vi "Simple main.vi"() -> ()   [LabVIEW 2021]
doc: "Use this template to build a simple state machine design pattern. Each state executes code and determines which state to transition to."
uses:
  controls/Data.ctl
  controls/State.ctl
  <instrlib>/Lake Shore 350/Lake Shore 350.lvlib
  <instrlib>/Keithley 2450/Keithley 2450.lvlib
panel:
  in  "Two way":bool
  out "Since last point (s)":dbl caption="Elapsed Time (s)"
  in  "Data spacing":enum16{"Log", "Quadratic", "Cubic", "Linear"}(ring)
  in  "Time Target (s)":dbl=3600.0 format="%#_13g"
  in  "Number of points":i32=390
  out "Progress %":dbl(slide) caption="Horizontal Pointer Slide" scale=0.0..100.0
  out "Data":T1
  in  "Start point":dbl
  in  "End point":dbl
  in  "Use second SMUs":bool
  in  "Stop btn":bool
  in  "Start btn":bool
  in  "Instruments":T2 {"SMU 2"."Last updated" format="%<%H:%M:%S>T"; "SMU 1"."Last updated" format="%<%H:%M:%S>T"; "TC"."Last updated" format="%<%H:%M:%S>T"}
  in  "End btn":bool
  out "Actual temperature chart":dbl[](graph)
  out "Rezistance graph":cluster{dbl[], dbl[]}[](graph)
  out "Message logs":string[](array[string])
  # "T=1,6*exp(0,0135*n)     where n is N in <1,"
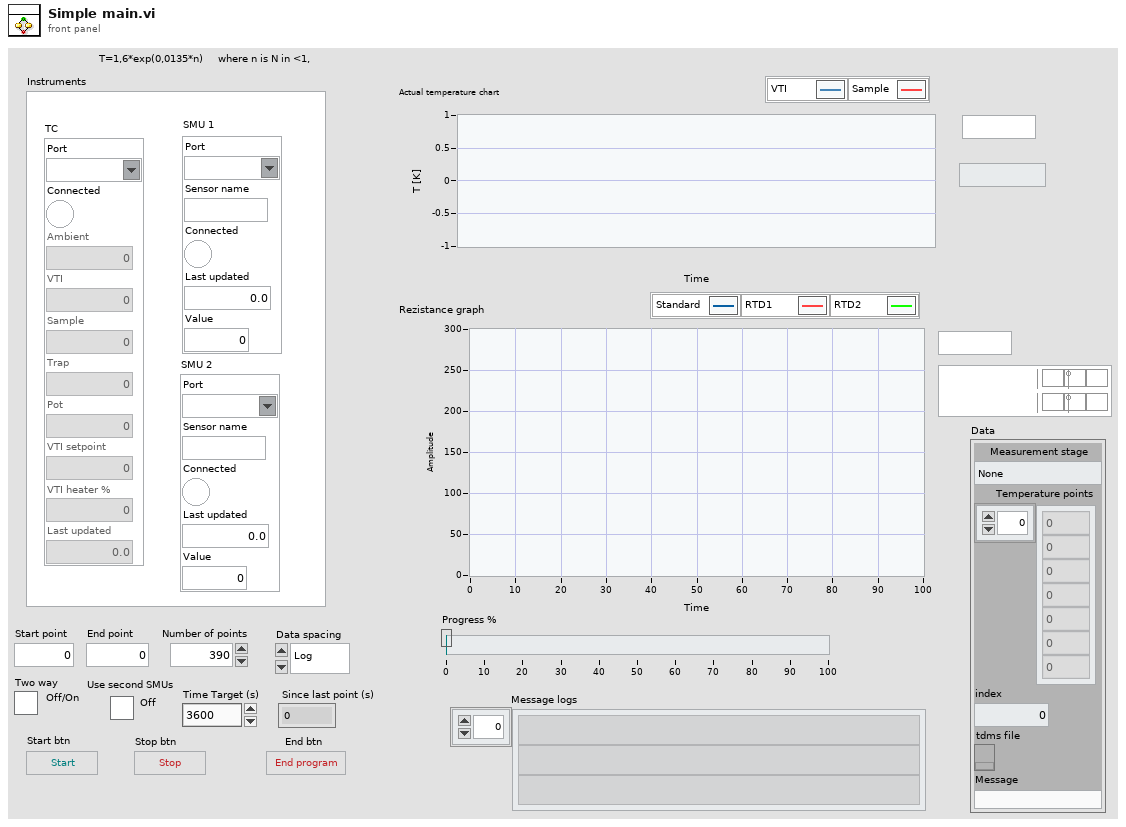
[diagram p1: front panel]
types:
  T1 = typedef "Data.ctl" = cluster{"Measurement stage":enum16{"None", "Wait to start", "Stage 1", "Interstage", "Stage 2", "Stopping"}, "Temperature points":dbl[], "index":i32, "tdms file":refnum<k34>, "Message":string}
  T2 = cluster{"TC":cluster{"Port":refnum<visa-resource-name>, "Connected":bool, "Ambient":dbl, "VTI":dbl, "Sample":dbl, "Trap":dbl, "Pot":dbl, "VTI setpoint":dbl, "VTI heater %":dbl, "Last updated":dbl}, "SMU 1":cluster{"Port":refnum<visa-resource-name>, "Sensor name":string, "Connected":bool, "Last updated":dbl, "Value":dbl}, "SMU 2":cluster{"Port":refnum<visa-resource-name>, "Sensor name":string, "Connected":bool, "Last updated":dbl, "Value":dbl}}
  T3 = typedef "State.ctl" = enum16{"Initialize", "Connect to TC", "Disconnect TC", "Connect to SMU", "Disconnect SMU ", "Set TC", "Read TC", "Set SMU", "Read SMU", "Wait for Event", "Start measurement", "Save datapoint", "End measurement", "Stop program"}
  T4 = enum16{"None", "Wait to start", "Stage 1", "Interstage", "Stage 2", "Stopping"}
  T5 = cluster{"Baud Rate":u32, "Parity":u16, "Data Bits":u16, "Stop Bits":u16, "Flow Control":u16}
  T6 = cluster{"Port":refnum<visa-resource-name>, "Sensor name":string, "Connected":bool, "Last updated":dbl, "Value":dbl}
  T7 = cluster{"Port":refnum<visa-resource-name>, "Connected":bool, "Ambient":dbl, "VTI":dbl, "Sample":dbl, "Trap":dbl, "Pot":dbl, "VTI setpoint":dbl, "VTI heater %":dbl, "Last updated":dbl}
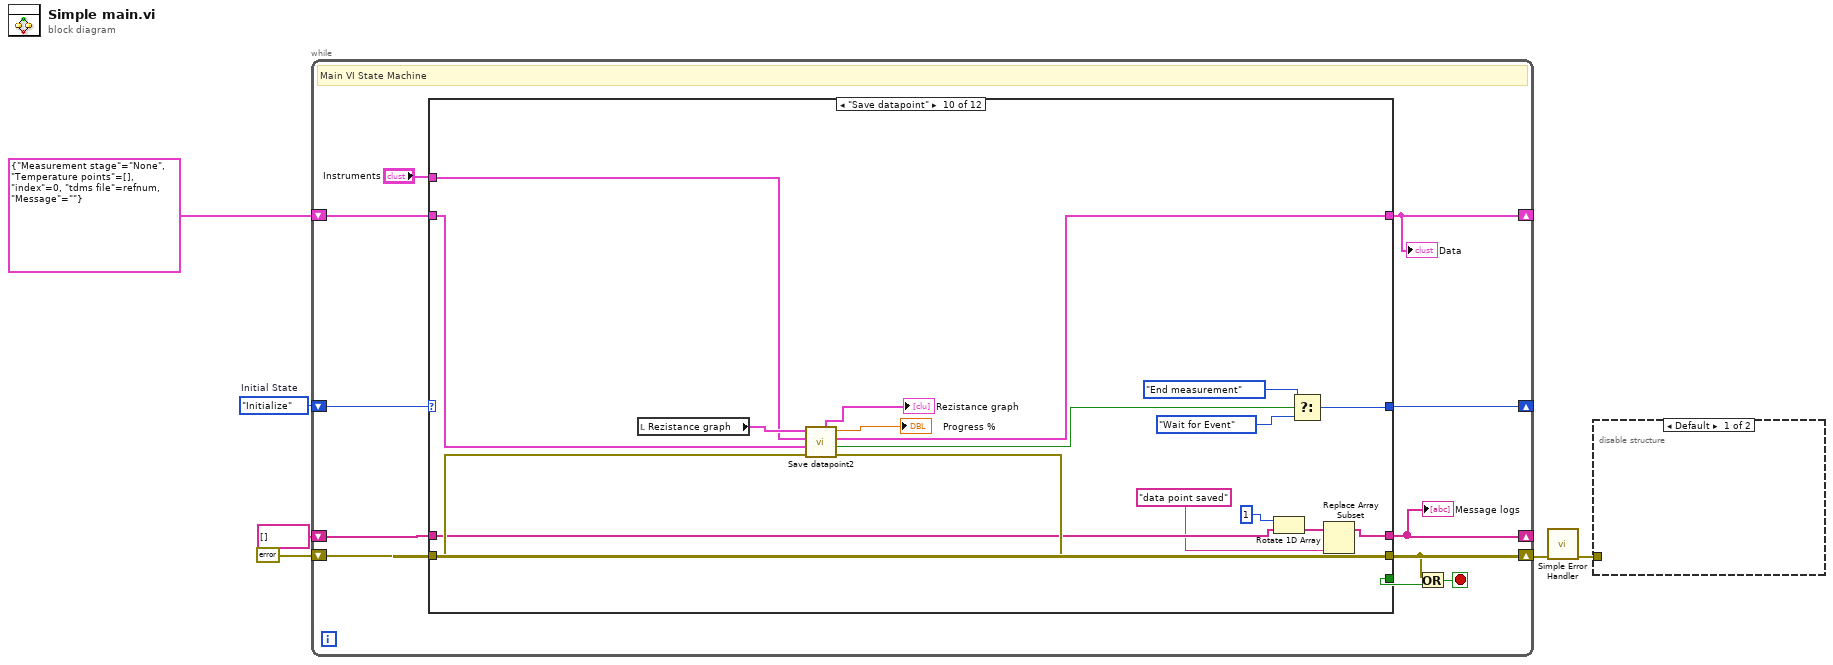
[diagram p0: block diagram]
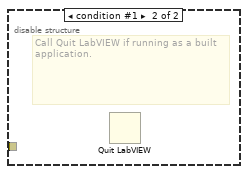
[diagram p2: hidden frame]
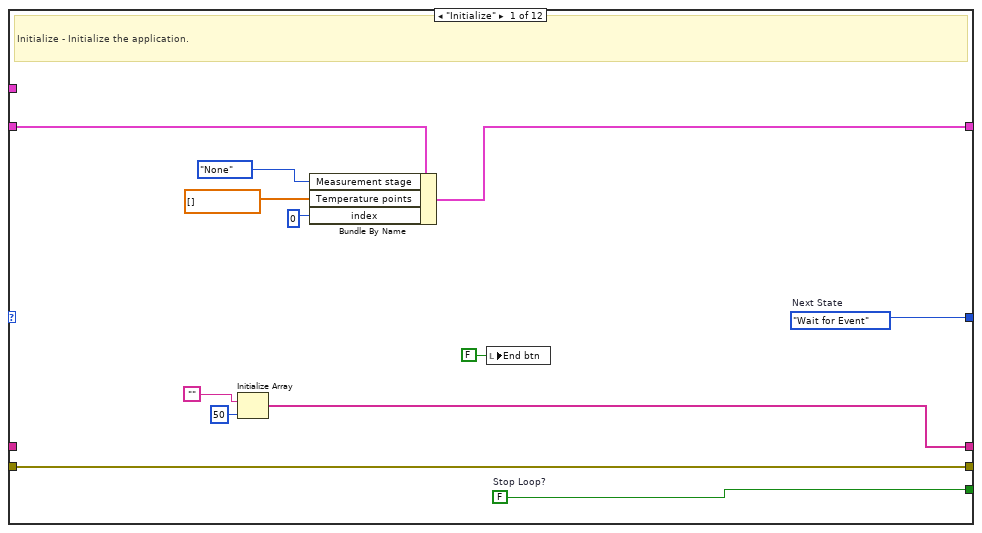
[diagram p3: hidden frame]
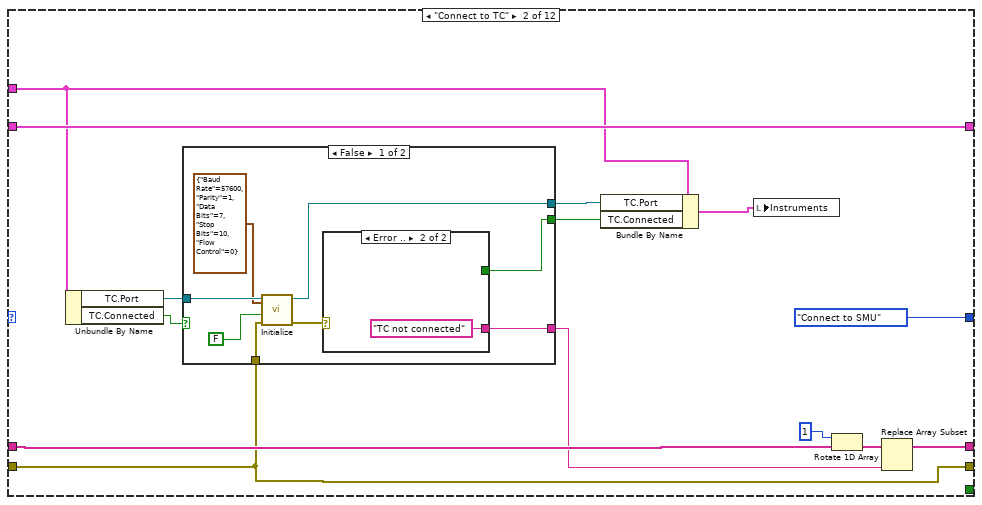
[diagram p4: hidden frame]
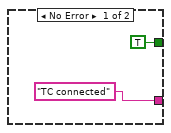
[diagram p5: hidden frame]
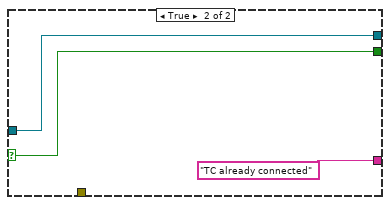
[diagram p6: hidden frame]
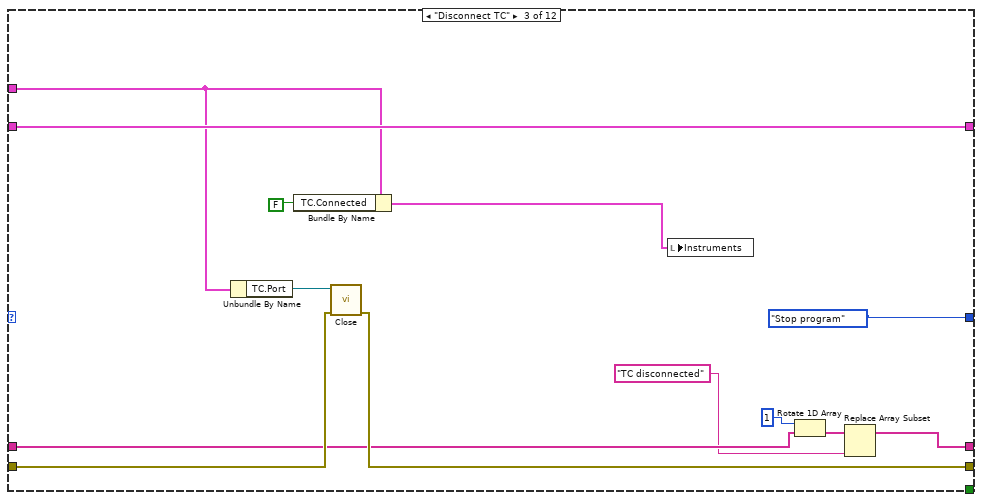
[diagram p7: hidden frame]
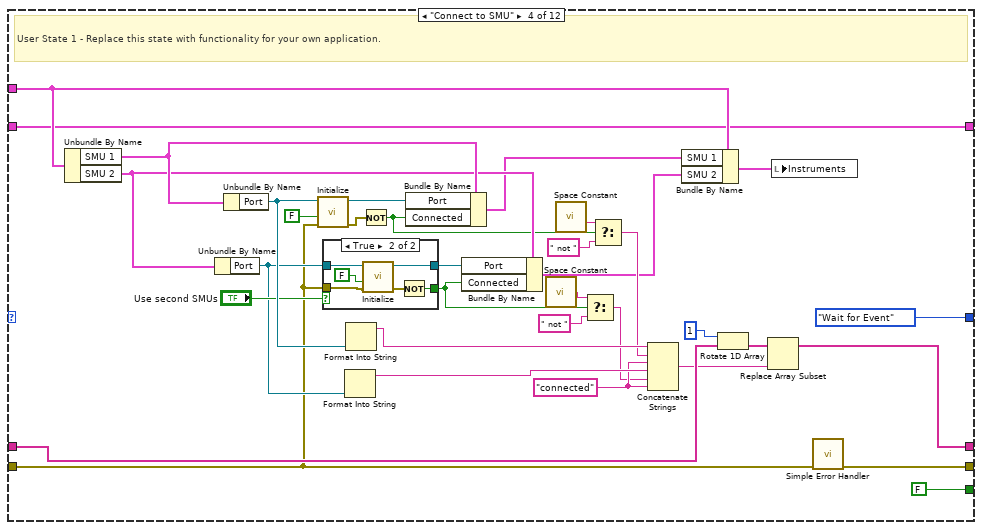
[diagram p8: hidden frame]
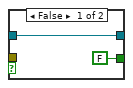
[diagram p9: hidden frame]
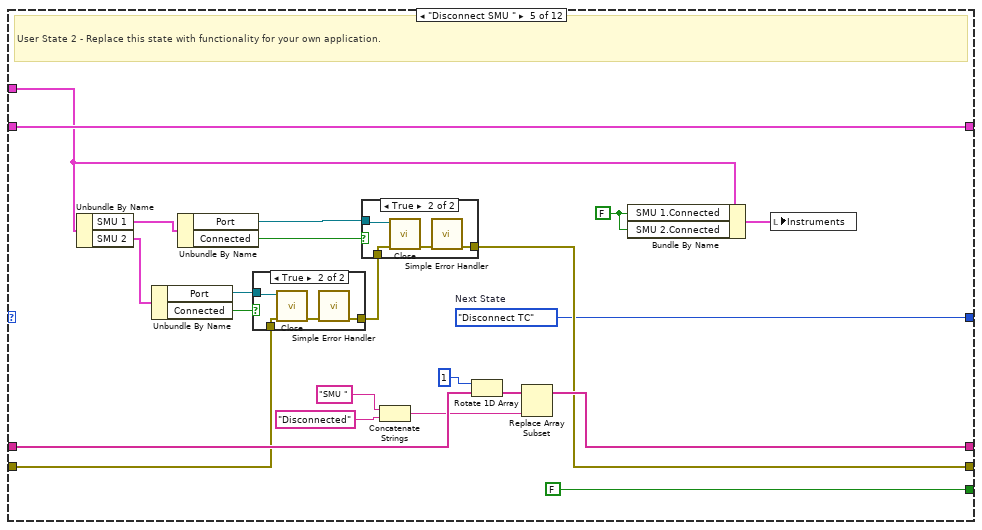
[diagram p10: hidden frame]
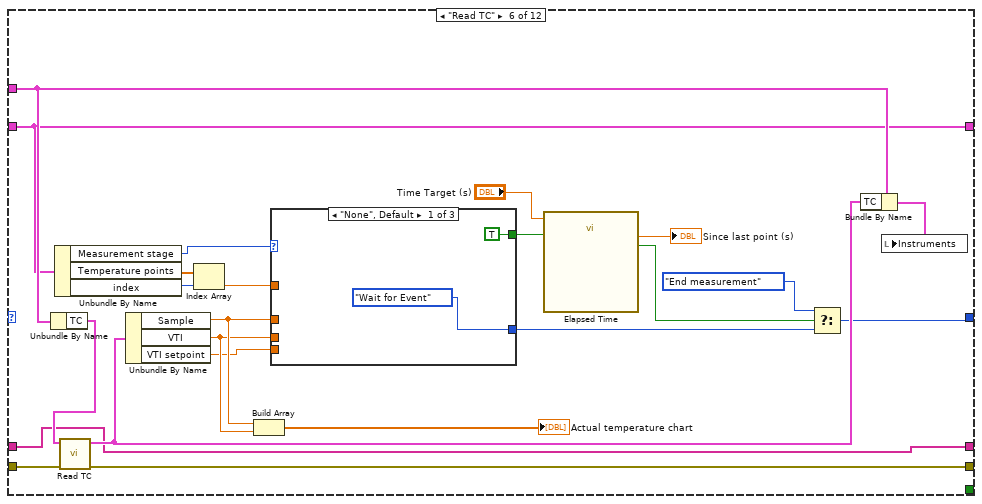
[diagram p13: hidden frame]
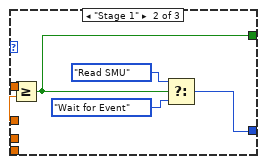
[diagram p14: hidden frame]
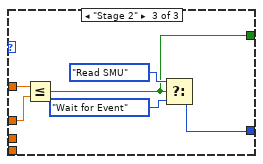
[diagram p15: hidden frame]
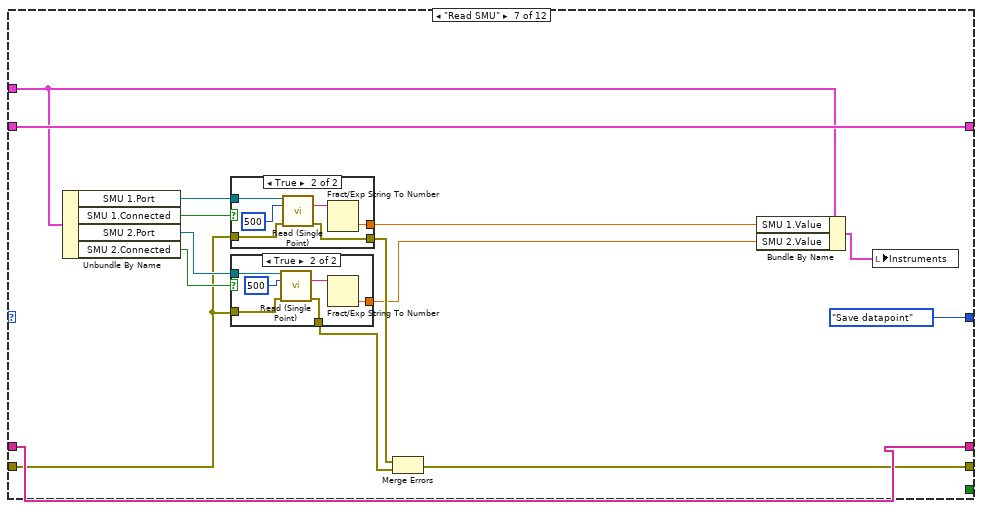
[diagram p16: hidden frame]
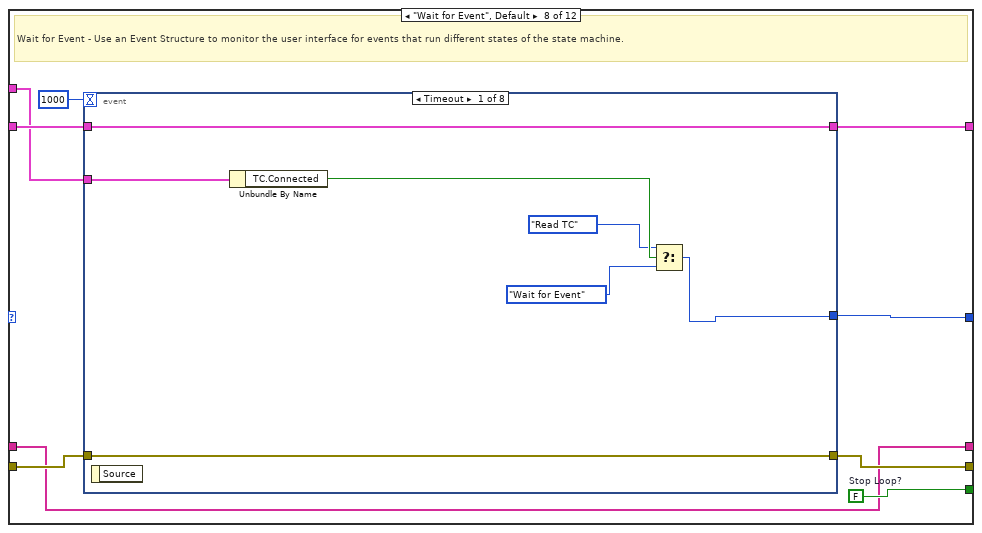
[diagram p19: hidden frame]
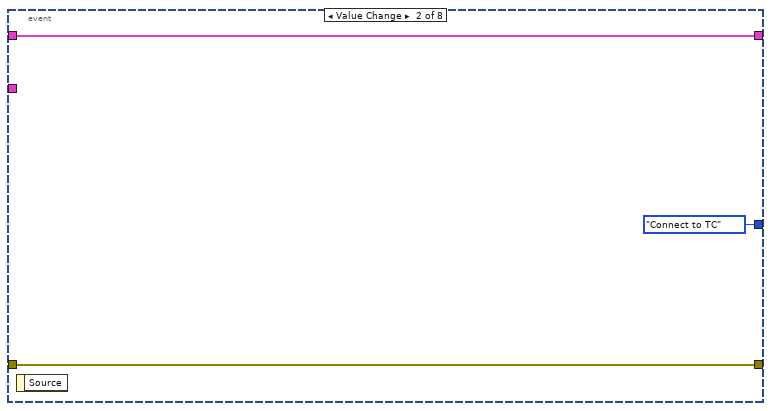
[diagram p20: hidden frame]
diagram:
  w6 = State."Initialize"  # Initial State
  n1 = while {
    shift-right: [w16] -> _
    shift-left: w6 -> [w17]
    shift-right: [w14] -> _
    shift-left: T1 {"Measurement stage"=enum."None", "Temperature points"=[], "index"=0, "tdms file"=refnum, "Message"=""} ("Data") -> [w15]
    shift-right: [w10] -> w3
    shift-left: errorcluster {"status"=FALSE, "code"=0, "source"=""} ("error constant") -> [w13]
    shift-right: [w8] -> _
    shift-left: string[] [] -> [w9]
    stop <- w11 stop-if-true
    # "Main VI State Machine"
    n2 = case shown="\"Save datapoint\"" w17 {
      tunnel: [w29 State."Connect to SMU" ("f") State."Stop program" ("(Value Not Used)") State."Wait for Event" ("(Value Not Used)") w116 w150 State."Save datapoint" ("(Value Not Used)") w219 State."Read TC" ("(Value Not Used)") w291 w318 w338] -> w16
      tunnel: [w28 _ _ FALSE ("Stop Loop?") FALSE ("Stop Loop?") _ _ w218 _ _ _ w336] -> w12
      tunnel: w15 -> [w27 w43 w70 w74 w133 w163 w194 w217 w266 w293 w317 w337]
      tunnel: [w26 w43 w70 w74 w133 w163 w194 w216 w276 w286 w309 w337] -> w14
      tunnel: w13 -> [w25 w35 w69 w72 w118 w166 w188 w215 w270 w287 w303 w335]
      tunnel: [w25 w35 w67 w103 w123 w167 w187 w214 w269 w288 w304 w335] -> w10
      tunnel: "Instruments" -> [_ w34 w65 w94 w114 w164 w193 w211 w275 w277 _ _]
      tunnel: [w19 w37 w61 w98 w126 w147 w195 w212 w261 w279 w299 w332] -> w8
      tunnel: w9 -> [_ w40 w60 w100 w128 w147 w195 w212 w260 w280 w300 w334]
      frame "Initialize" {
        w28 = FALSE  # Stop Loop?
        w29 = State."Wait for Event"  # Next State
        # "Initialize - Initialize the application."
        n3 = Initialize Array("", 50 ("dimension size")) -> (w19:string[])
        n4 = Bundle By Name(cluster=w27, "Measurement stage"=T4."None", "Temperature points"=dbl[] [], "index"=0) -> (w26:T1)
        n5 = local write "End btn"(FALSE ("End btn")) -> ()
      }
      frame "Connect to TC" {
        n6 = Unbundle By Name(w34) -> ("TC.Port"=w42:refnum<visa-resource-name>, "TC.Connected"=w36:bool)
        n7 = case shown="False" w36 {
          selector: w36 -> [_ w56]
          tunnel: w42 -> [w51 w57]
          tunnel: w35 -> [w49 _]
          tunnel: [w48 w57] -> w33
          tunnel: [w44 w56] -> w32
          tunnel: [w45 "TC already connected" ("f")] -> w31
          frame False {
            n8 = call <instrlib>:"Initialize.vi"("Serial Configuration"=T5 {"Baud Rate"=57600, "Parity"=1, "Data Bits"=7, "Stop Bits"=10, "Flow Control"=0}, "error in (no error)"=w49, "Reset (True)"=FALSE, "VISA resource name"=w51) -> ("error out"=w46:errorcluster, "VISA resource name out"=w48:refnum<visa-resource-name>)  [unwired: 6 in]
            n9 = case shown="Error .." w46 {
              tunnel: ["TC connected" "TC not connected" ("f")] -> w45
              tunnel: [TRUE _] -> w44
              frame No Error {
              }
              frame Error {
              }
            }
          }
          frame True {
          }
        }
        n10 = Bundle By Name(cluster=w34, "TC.Port"=w33, "TC.Connected"=w32) -> (w30:T2)
        n11 = local write "Instruments"(w30) -> ()
        n12 = Rotate 1D Array(1:w40, 2:1 ("n")) -> (0:w39:string[])
        n13 = Replace Array Subset(array=w39, new element=w31) -> (w37:string[])  [unwired: 1 in]
      }
      frame "Disconnect TC" {
        n14 = Unbundle By Name(w65) -> ("TC.Port"=w68:refnum<visa-resource-name>)
        n15 = Bundle By Name(cluster=w65, "TC.Connected"=FALSE) -> (w58:T2)
        n16 = call <instrlib>:"Close.vi"("error in (no error)"=w69, "VISA resource name"=w68) -> ("error out"=w67:errorcluster)  [unwired: 9 in]
        n17 = local write "Instruments"(w58) -> ()
        n18 = Rotate 1D Array(1:w60, 2:1 ("n")) -> (0:w63:string[])
        n19 = Replace Array Subset(array=w63, new element="TC disconnected") -> (w61:string[])  [unwired: 1 in]
      }
      frame "Connect to SMU" {
        w82 = "connected"
        # "User State 1 - Replace this state with functionality for your own application."
        n20 = Unbundle By Name(w94) -> ("SMU 1"=w93:T6, "SMU 2"=w91:T6)
        n21 = Unbundle By Name(w91) -> ("Port"=w86:refnum<visa-resource-name>)
        n22 = Unbundle By Name(w93) -> ("Port"=w97:refnum<visa-resource-name>)
        n23 = call <instrlib>:"Initialize.vi"("error in (no error)"=w72, "Reset (True)"=FALSE, "VISA resource name"=w97) -> ("error out"=w75:errorcluster, "VISA resource name out"=w92:refnum<visa-resource-name>)  [unwired: 7 in]
        n24 = case shown="True" "Use second SMUs" {
          tunnel: w86 -> [w106 w111]
          tunnel: [w106 w110] -> w90
          tunnel: [FALSE w109] -> w78
          tunnel: w72 -> [_ w107]
          frame False {
          }
          frame True {
            n25 = call <instrlib>:"Initialize.vi"("error in (no error)"=w107, "Reset (True)"=FALSE, "VISA resource name"=w111) -> ("error out"=w108:errorcluster, "VISA resource name out"=w110:refnum<visa-resource-name>)  [unwired: 7 in]
            n26 = Not(x=w108) -> (.not. x?=w109:bool)
          }
        }
        n27 = Format Into String(w86) -> (resulting string=w83:string)  [unwired: 3 in, 1 out]
        n28 = Format Into String(w97) -> (resulting string=w85:string)  [unwired: 3 in, 1 out]
        n29 = Not(x=w75) -> (.not. x?=w87:bool)
        n30 = Bundle By Name(cluster=w93, "Port"=w92, "Connected"=w87) -> (w76:T6)
        n31 = Bundle By Name(cluster=w91, "Port"=w90, "Connected"=w78) -> (w77:T6)
        n32 = call <vilib>:"Space Constant.vi"() -> ("String"=w81:string)
        n33 = call <vilib>:"Space Constant.vi"() -> ("String"=w88:string)
        n34 = Select(t=w81, s=w78, f=" not ") -> (s? t:f=w79:string)
        n35 = Select(t=w88, s=w87, f=" not ") -> (s? t:f=w84:string)
        n36 = Concatenate Strings(w85, w84, w82, w83, w79, w82) -> (w99:string)
        n37 = Bundle By Name(cluster=w94, "SMU 1"=w76, "SMU 2"=w77) -> (w71:T2)
        n38 = Rotate 1D Array(1:w100, 2:1 ("n")) -> (0:w102:string[])
        n39 = Replace Array Subset(array=w102, new element=w99) -> (w98:string[])  [unwired: 1 in]
        n40 = local write "Instruments"(w71) -> ()
        n41 = call <vilib>:"Simple Error Handler.vi"("error in (no error)"=w72) -> ("error out"=w103:errorcluster)  [unwired: 4 in, 4 out]
      }
      frame "Disconnect SMU " {
        w113 = FALSE
        w116 = State."Disconnect TC"  # Next State
        # "User State 2 - Replace this state with functionality for your own application."
        n42 = Unbundle By Name(w114) -> ("SMU 1"=w121:T6, "SMU 2"=w122:T6)
        n43 = Unbundle By Name(w122) -> ("Port"=w120:refnum<visa-resource-name>, "Connected"=w119:bool)
        n44 = Unbundle By Name(w121) -> ("Port"=w125:refnum<visa-resource-name>, "Connected"=w124:bool)
        n45 = case shown="True" w119 {
          tunnel: w120 -> [_ w139]
          tunnel: w118 -> [w135 w137]
          tunnel: [w135 w136] -> w117
          frame False {
          }
          frame True {
            n46 = call <instrlib>:"Close.vi"("error in (no error)"=w137, "VISA resource name"=w139) -> ("error out"=w138:errorcluster)  [unwired: 9 in]
            n47 = call <vilib>:"Simple Error Handler.vi"("error in (no error)"=w138) -> ("error out"=w136:errorcluster)  [unwired: 4 in, 4 out]
          }
        }
        n48 = case shown="True" w124 {
          tunnel: w125 -> [_ w144]
          tunnel: w117 -> [w140 w142]
          tunnel: [w140 w141] -> w123
          frame False {
          }
          frame True {
            n49 = call <instrlib>:"Close.vi"("error in (no error)"=w142, "VISA resource name"=w144) -> ("error out"=w143:errorcluster)  [unwired: 9 in]
            n50 = call <vilib>:"Simple Error Handler.vi"("error in (no error)"=w143) -> ("error out"=w141:errorcluster)  [unwired: 4 in, 4 out]
          }
        }
        n51 = Concatenate Strings("SMU ", "Disconnected") -> (w127:string)
        n52 = Rotate 1D Array(1:w128, 2:1 ("n")) -> (0:w130:string[])
        n53 = Replace Array Subset(array=w130, new element=w127) -> (w126:string[])  [unwired: 1 in]
        n54 = Bundle By Name(cluster=w114, "SMU 1.Connected"=w113, "SMU 2.Connected"=w113) -> (w115:T2)
        n55 = local write "Instruments"(w115) -> ()
      }
      frame "Read TC" {
        n56 = Unbundle By Name(w164) -> ("TC"=w165:T7)
        n57 = Unbundle By Name(w163) -> ("Measurement stage"=w160:T4, "Temperature points"=w162:dbl[], "index"=w161:i32)
        n58 = call "Read TC.vi"("error in (no error)"=w166, "TC in"=w165) -> ("error out"=w167:errorcluster, "TC out"=w157:T7)  [unwired: 8 in]
        n59 = Unbundle By Name(w157) -> ("Sample"=w154:dbl, "VTI"=w152:dbl, "VTI setpoint"=w151:dbl)
        n60 = Index Array(array=w162, index=w161) -> (element=w158:dbl)
        n61 = Build Array(w154, w152) -> (→"Actual temperature chart":dbl[])
        n62 = case shown="\"None\", Default" w160 {
          tunnel: [State."Wait for Event" ("(Value Not Used)") w174 w180] -> w159
          tunnel: w158 -> [_ w172 w178]
          tunnel: w154 -> [_ w171 w177]
          tunnel: [TRUE w170 w176] -> w156
          tunnel: w152 -> [_ _ _]
          tunnel: w151 -> [_ _ _]
          frame "None", Default {
          }
          frame "Stage 1" {
            n63 = Greater Or Equal?(x=w172, y=w171) -> (x >= y?=w170:bool)
            n64 = Select(t=State."Read SMU", s=w170, f=State."Wait for Event") -> (s? t:f=w174:T3)
          }
          frame "Stage 2" {
            n65 = Less Or Equal?(x=w178, y=w177) -> (x <= y?=w176:bool)
            n66 = Select(t=State."Read SMU", s=w176, f=State."Wait for Event") -> (s? t:f=w180:T3)
          }
        }
        n67 = call "Elapsed Time"("Time Target (s)"="Time Target (s)", "Reset"=w156) -> ("Elapsed Time (s)"=→"Since last point (s)":dbl, "Time has Elapsed"=w149:bool)  [unwired: 10 in, 6 out]
        n68 = Select(t=State."End measurement", s=w149, f=w159) -> (s? t:f=w150:T3)
        n69 = Bundle By Name(cluster=w164, "TC"=w157) -> (w145:T2)
        n70 = local write "Instruments"(w145) -> ()
      }
      frame "Read SMU" {
        n71 = Unbundle By Name(w193) -> ("SMU 1.Port"=w191:refnum<visa-resource-name>, "SMU 1.Connected"=w192:bool, "SMU 2.Port"=w190:refnum<visa-resource-name>, "SMU 2.Connected"=w189:bool)
        n72 = case shown="True" w192 {
          tunnel: w191 -> [_ w208]
          tunnel: w188 -> [w204 w207]
          tunnel: [w204 w206] -> w186
          tunnel: [_ w205] -> w184
          frame False {
          }
          frame True {
            n73 = call <instrlib>:"Read (Single Point).vi"("VISA resource name"=w208, "Timeout (10000 ms)"=500, "error in (no error)"=w207) -> ("Data out"=w209:string, "error out"=w206:errorcluster)  [unwired: 10 in, 1 out]
            n74 = Fract/Exp String To Number(string=w209) -> (number=w205:dbl)  [unwired: 3 in, 1 out]
          }
        }
        n75 = case shown="True" w189 {
          tunnel: w190 -> [_ w201]
          tunnel: w188 -> [w197 w200]
          tunnel: [w197 w199] -> w185
          tunnel: [_ w198] -> w183
          frame False {
          }
          frame True {
            n76 = call <instrlib>:"Read (Single Point).vi"("VISA resource name"=w201, "Timeout (10000 ms)"=500, "error in (no error)"=w200) -> ("Data out"=w202:string, "error out"=w199:errorcluster)  [unwired: 10 in, 1 out]
            n77 = Fract/Exp String To Number(string=w202) -> (number=w198:dbl)  [unwired: 3 in, 1 out]
          }
        }
        n78 = Merge Errors(w186, w185) -> (w187:errorcluster)
        n79 = Bundle By Name(cluster=w193, "SMU 1.Value"=w184, "SMU 2.Value"=w183) -> (w182:T2)
        n80 = local write "Instruments"(w182) -> ()
      }
      frame "Wait for Event", Default {
        w218 = FALSE  # Stop Loop?
        # "Wait for Event - Use an Event Structure to monitor the user interface for events that run different states of the state machine."
        n81 = event shown="[0] Timeout" {
          selector: _ -> [_ _ _ _ _ _ _ _]
          dyn-events: _ -> [_ _ _ _ _ _ _ _]
          timeout: 1000 -> [_ _ _ _ _ _ _ _]
          tunnel: [w222 State."Connect to TC" ("Next State") State."Connect to SMU" ("Next State") w233 w243 w248 State."End measurement" ("Next State") w254] -> w219
          tunnel: w217 -> [w225 w229 w232 w238 w242 w247 w251 w253]
          tunnel: [w225 w229 w232 w238 w241 w246 w251 w253] -> w216
          tunnel: w215 -> [w226 w228 w231 w237 w239 w244 w250 w252]
          tunnel: [w226 w228 w231 w237 w239 w244 w250 w252] -> w214
          tunnel: w211 -> [w220 _ _ _ _ _ _ _]
          event Timeout {
            n82 = event-data() -> ()  [unwired: 1 in, 1 out]
            n83 = Unbundle By Name(w220) -> ("TC.Connected"=w224:bool)
            n84 = Select(t=State."Read TC" ("Next State"), s=w224, f=State."Wait for Event") -> (s? t:f=w222:T3)
          }
          event "Instruments.TC.Port": Value Change {
            n85 = event-data() -> ()  [unwired: 1 in, 1 out]
          }
          event "Instruments.SMU 1.Port", "Instruments.SMU 2.Port": Value Change {
            n86 = event-data() -> ()  [unwired: 1 in, 1 out]
          }
          event "Use second SMUs": Value Change {
            n87 = event-data() -> ("NewVal"=w234:bool)  [unwired: 1 in, 1 out]
            n88 = Select(t=State."Connect to SMU" ("Next State"), s=w234, f=State."Disconnect SMU " ("Next State")) -> (s? t:f=w233:T3)
          }
          event "Start point": Value Change {
            w243 = State."Set TC"  # Next State
            n89 = event-data() -> ()  [unwired: 1 in, 1 out]
            n90 = Bundle By Name(cluster=w242, "Message"="Running User State 1" ("Running User State 1")) -> (w241:T1)
          }
          event "Start btn": Value Change {
            w248 = State."Start measurement"  # Next State
            n91 = event-data() -> ()  [unwired: 1 in, 1 out]
            n92 = Bundle By Name(cluster=w247, "Message"="Start" ("Running User State 2")) -> (w246:T1)
          }
          event "Stop btn": Value Change {
            n93 = event-data() -> ()  [unwired: 1 in, 1 out]
          }
          event "End btn": Value Change {
            w254 = State."Connect to SMU"  # Next State
            n94 = event-data() -> ()  [unwired: 1 in, 1 out]
          }
        }
      }
      frame "Start measurement" {
        n95 = Unbundle By Name(w275) -> ("SMU 1.Sensor name"=w256:string, "SMU 2.Sensor name"=w255:string, "TC.Ambient"=w271:dbl)
        n96 = call "Generate tmp points.vi"("Type"="Data spacing", "Number of points"="Number of points", "End point"="End point", "Start point"="Start point") -> ("Array"=w272:dbl[])  [unwired: 7 in]
        n97 = call "Create meas file with date.vi"("Start point"="Start point", "Ambient T"=w271, "End point"="End point", "error in (no error)"=w270, "Array"=w272, "Sensor 2 name"=w255, "Sensor 1 name"=w256) -> ("error out"=w269:errorcluster, "tdms file out"=w268:refnum<k34>)  [unwired: 3 in]
        n98 = local write "Rezistance graph"(cluster{dbl[], dbl[]}[] [] ("Rezistance graph")) -> ()
        n99 = invoke on="Actual temperature chart" class="WFChart (strict)" method="Reinit To Default"() -> ()  [unwired: 3 in, 3 out]
        n100 = Bundle By Name(cluster=w266, "Temperature points"=w272, "tdms file"=w268, "Measurement stage"=T4."Stage 1") -> (w276:T1)
        n101 = Rotate 1D Array(1:w260, 2:1 ("n")) -> (0:w263:string[])
        n102 = Replace Array Subset(array=w263, new element="Preparing to start measurement.") -> (w261:string[])  [unwired: 1 in]
      }
      frame "Save datapoint" {
        n103 = local read "Rezistance graph"() -> (w284:cluster{dbl[], dbl[]}[])
        n104 = call "Save datapoint2.vi"("error in (no error)"=w287, "Data in"=w293, "Instruments"=w277, "graph data in"=w284) -> ("error out"=w288:errorcluster, "Is complete"=w289:bool, "Data out"=w286:T1, "Progress %"=→"Progress %":dbl, "Graph data out"=→"Rezistance graph":cluster{"Array":dbl[], "Array":dbl[]}[])  [unwired: 3 in]
        n105 = Rotate 1D Array(1:w280, 2:1 ("n")) -> (0:w282:string[])
        n106 = Select(t=State."End measurement" ("(Value Not Used)"), s=w289, f=State."Wait for Event") -> (s? t:f=w291:T3)
        n107 = Replace Array Subset(array=w282, new element="data point saved") -> (w279:string[])  [unwired: 1 in]
      }
      frame "End measurement" {
        n108 = Unbundle By Name(w317) -> ("Measurement stage"=w297:T4, "Temperature points"=w310:dbl[], "tdms file"=w313:refnum<k34>)  [unwired: 1 out]
        n109 = Format Into String(w297) -> (resulting string=w295:string)  [unwired: 3 in, 1 out]
        n110 = Concatenate Strings(w295, " finished") -> (w296:string)
        n111 = Equal?(x=w297, y=T4."Stage 1") -> (x = y?=w316:bool)
        n112 = TDMS Close(8:w303, 11:w313) -> (0:w311:errorcluster, 3:w312:path)
        n113 = And(x=w316, y="Two way") -> (x .and. y?=w314:bool)
        n114 = case shown="False" w314 {
          tunnel: [State."Wait for Event" ("(Value Not Used)") State."Set TC" ("(Value Not Used)")] -> w318
          tunnel: w312 -> [_ w328]
          tunnel: w311 -> [w321 w327]
          tunnel: w310 -> [_ w326]
          tunnel: [T4."None" ("y") T4."Stage 2" ("y")] -> w308
          tunnel: [_ w324] -> w307
          tunnel: [_ w323] -> w305
          tunnel: [w321 w322] -> w304
          frame False {
          }
          frame True {
            n115 = Reverse 1D Array(array=w326) -> (reversed array=w324:dbl[])
            n116 = TDMS Open(8:w327, 11:w328) -> (0:w322:errorcluster, 3:w323:refnum<k34>)  [unwired: 5 in]
          }
        }
        n117 = Bundle By Name(cluster=w317, "Measurement stage"=w308, "Temperature points"=w307, "index"=0, "tdms file"=w305) -> (w309:T1)
        n118 = Rotate 1D Array(1:w300, 2:1 ("n")) -> (0:w302:string[])
        n119 = Replace Array Subset(array=w302, new element=w296) -> (w299:string[])  [unwired: 1 in]
      }
      frame "Stop program" {
        w336 = TRUE  # Stop Loop?
        w338 = State."Stop program"  # (Value Not Used)
        # "#CodeNeeded - Add any required cleanup code here."
        # "The state value is not used here since this is the last iteration of the state machine loop."
        # "Exit - Exit the application."
        n120 = Rotate 1D Array(1:w334, 2:1 ("n")) -> (0:w333:string[])
        n121 = Replace Array Subset(array=w333, new element="Program stopped") -> (w332:string[])  [unwired: 1 in]
      }
    }
    "Message logs" <- w8
    "Data" <- w14
    n122 = Or(x=w10, y=w12) -> (x .or. y?=w11:bool)
  }
  n123 = call <vilib>:"Simple Error Handler.vi"("error in (no error)"=w3) -> ("error out"=w2:errorcluster)  [unwired: 4 in, 4 out]
  n124 = disable-structure shown="Default" {
    disable-tunnel: w2 -> [_ _]
    frame condition #0 (active) {
    }
    frame condition #1 {
      # "Call Quit LabVIEW if running as a built application."
      n125 = Quit LabVIEW() -> ()  [unwired: 1 in]
    }
  }
